vi "Read Single Point.vi"(8 "error in (no error)":errorcluster, 11 "Agilent 34401a in":refnum<class "Agilent 34401a.lvclass">) -> (0 "error out":errorcluster, 2 "Measurement":dbl, 3 "Agilent 34401a out":refnum<class "Agilent 34401a.lvclass">)   [LabVIEW 2026, in "Agilent 34401a.lvclass"]
uses:
  Agilent 34401a.lvclass
  Agilent 34401a.lvclass/Agilent 34401a.ctl
  <instrlib>/Agilent 34401/Public/Data/Read (Single Point).vi
  <instrlib>/Agilent 34401/Agilent 34401.lvlib
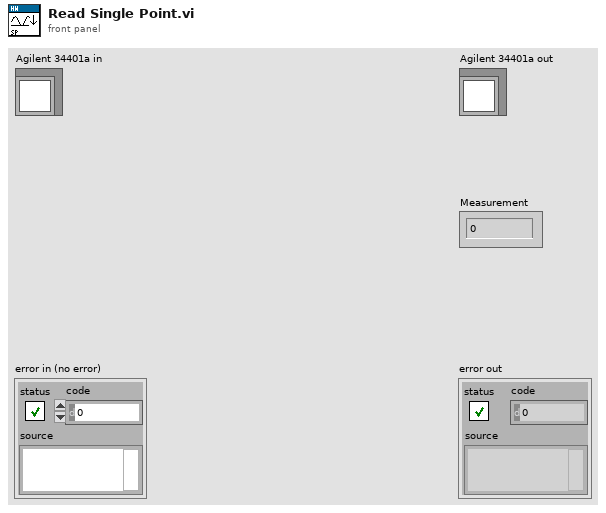
[diagram p1: front panel]
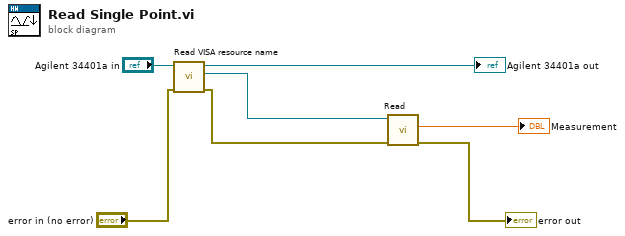
[diagram p0: block diagram]
diagram:
  n1 = call "Read VISA resource name.vi"("error in (no error)"="error in (no error)", "Agilent 34401a in"="Agilent 34401a in") -> ("error out"=w2:errorcluster, "VISA resource name"=w3:refnum<visa-resource-name>, "Agilent 34401a out"=→"Agilent 34401a out":refnum<class "Agilent 34401a.lvclass">)  [unwired: 7 in]
  n2 = call-poly <instrlib>:"Read.vi"("error in (no error)"=w2, "VISA resource name"=w3) -> ("error out"=→"error out":errorcluster, "Measurement"=→"Measurement":dbl)  [unwired: 7 in, 1 out]
